vi "UIProccessJoysticks.vi"(10 "Axes":dbl[](array[numeric])) -> ()   [LabVIEW 2014, in "UILib.lvlib"]
uses:
  UILib.lvlib
  ChassisLib/ChassisLib.lvlib
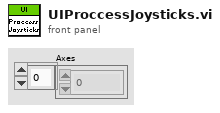
[diagram p1: front panel]
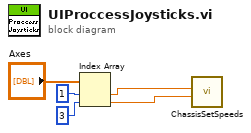
[diagram p0: block diagram]
diagram:
  n1 = Index Array(array="Axes", index #1=1 ("index"), index #2=3 ("index")) -> (element #1=w2:dbl, element #2=w1:dbl)
  n2 = call "ChassisSetSpeeds.vi"("DriveSpeedRight"=w1, "DriveSpeedLeft"=w2) -> ()  [unwired: 10 in]
